vi "curve-extract-gaussian fitting_sub.vi"(0 "X array":dbl[](array[numeric]), 1 "Y array":dbl[](array[numeric]), 2 "index":i32, 3 "length":i32) -> (5 "X subarray":dbl[](array[numeric]), 6 "Y subarray":dbl[](array[numeric]), 7 "BG_extracted":dbl[](array[numeric]), 8 "Best Gaussian Fit":dbl[](array[numeric]), 9 "amplitude":dbl, 10 "center":dbl)   [LabVIEW 2021]
uses:
  <vilib>/Analysis/NI_AALPro.lvlib
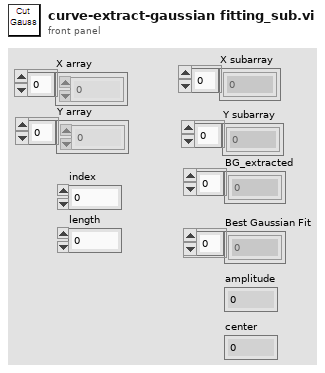
[diagram p1: front panel]
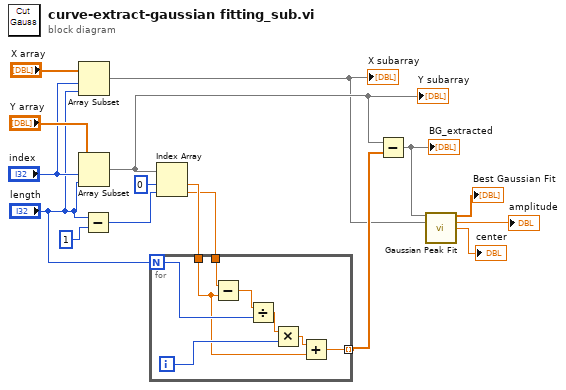
[diagram p0: block diagram]
diagram:
  n1 = Array Subset(array="X array", index="index", length="length") -> (w1:dbl[])
  "X subarray" <- w1
  n2 = Array Subset(array="Y array", index="index", length="length") -> (w10:dbl[])
  "Y subarray" <- w10
  n3 = Subtract(x="length", y=1) -> (x-y=w14:i32)
  n4 = Index Array(array=w10, index #1=0 ("index"), index #2=w14) -> (element #1=w13:dbl, element #2=w12:dbl)
  n5 = for {
    N: "length" -> [w22]
    tunnel: w13 -> [w18]
    tunnel: w12 -> [w24]
    tunnel: [w17] -> w11 mode=indexing
    i -> [w20]
    n6 = Subtract(x=w24, y=w18) -> (x-y=w23:dbl)
    n7 = Divide(x=w23, y=w22) -> (x/y=w21:dbl)
    n8 = Multiply(x=w21, y=w20) -> (x*y=w19:dbl)
    n9 = Add(x=w19, y=w18) -> (x+y=w17:dbl)
  }
  n10 = Subtract(x=w10, y=w11) -> (x-y=w5:dbl[])
  "BG_extracted" <- w5
  n11 = call <vilib>:"Gaussian Peak Fit.vi"("Y"=w5, "X"=w1) -> ("Best Gaussian Fit"=→"Best Gaussian Fit":dbl[], "amplitude"=→"amplitude":dbl, "center"=→"center":dbl)  [unwired: 7 in, 4 out]
